vi "Detector Close.vi"(8 "error in (no error)":errorcluster, 11 "PRIME Detector in":refnum<class "PRIME Detector.lvclass">) -> (0 "error out":errorcluster, 3 "PRIME Detector out":refnum<class "PRIME Detector.lvclass">)   [LabVIEW 2021, in "PRIME Detector.lvclass"]
uses:
  PRIME Detector.lvclass
  PRIME Detector.lvclass/PRIME Detector.ctl
  f8fde255-d984-4f84-9304-7df44634cede.vi
  Detector Class.lvclass
panel:
  out "Responses":string[](array[string])
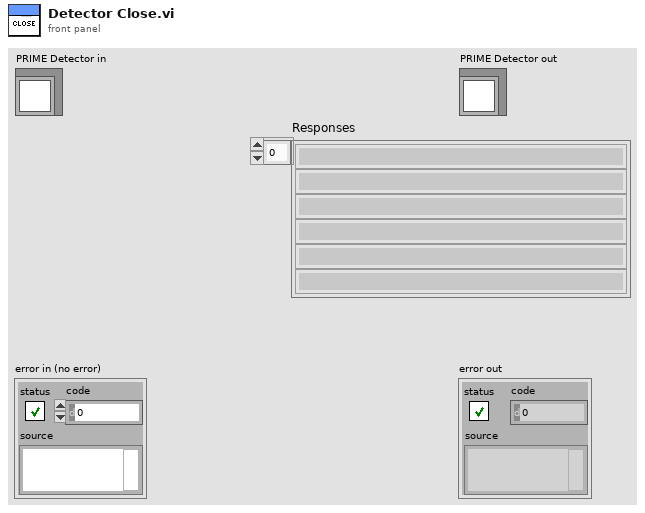
[diagram p1: front panel]
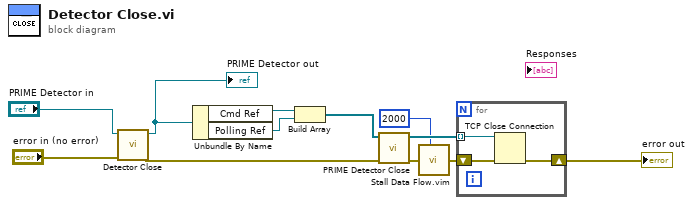
[diagram p0: block diagram]
diagram:
  n1 = call-parent "Detector Close.vi"("error in (no error)"="error in (no error)", "Detector Class in"="PRIME Detector in") -> ("error out"=w8:errorcluster, "Detector Class out"=w10:refnum<class "PRIME Detector.lvclass">)  [unwired: 8 in]
  "PRIME Detector out" <- w10
  n2 = Unbundle By Name(w10) -> ("Cmd Ref"=w5:refnum<k5>, "Polling Ref"=w4:refnum<k5>)
  n3 = Build Array(w5, w4) -> (w3:refnum<k5>[])
  n4 = call "PRIME Detector Close.vi"("error in (no error)"=w8, "connection ID"=w3) -> ("error out"=w6:errorcluster, "connection ID out"=w7:refnum<k5>[])  [unwired: 8 in]
  n5 = call "Stall Data Flow.vim"("value in"=w6, "milliseconds to wait"=u32 2000) -> ("value out"=w2:errorcluster)  [unwired: 1 out]
  n6 = for {
    tunnel: w7 -> [w14] mode=indexing
    shift-right: [w15] -> w9
    shift-left: w2 -> [w13]
    n7 = TCP Close Connection(connection ID=w14, error in (no error)=w13) -> (error out=w15:errorcluster)  [unwired: 1 in, 1 out]
  }
  "error out" <- w9
